vi "Historial de coordenadas.vi"(10 "Array":string[](array[string])) -> ()   [LabVIEW 2021]
panel:
  # "Lectura del arreglo de los cambios del setpoint"
  # "Elaborado por: Rodríguez Corona Ernesto \n04 de marzo del 2022"
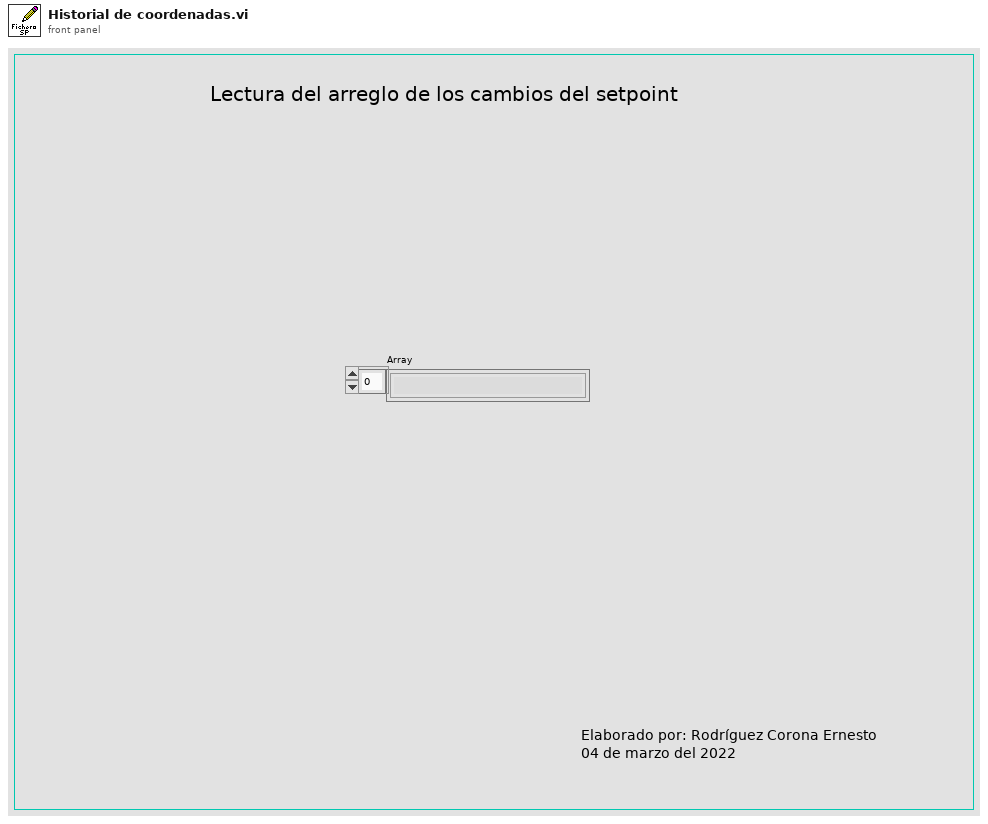
[diagram p1: front panel]
types:
  T1 = enum16{"open", "replace", "create", "open or create", "replace or create", "replace or create with confirmation"}
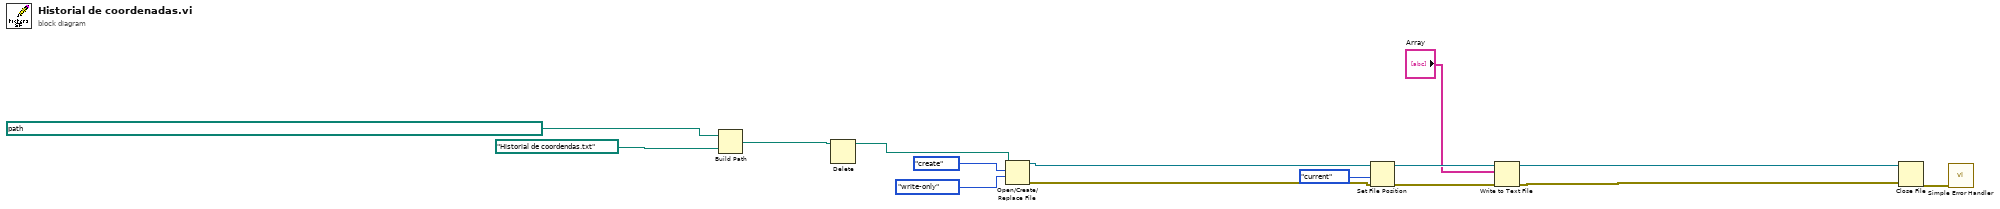
[diagram p0: block diagram]
diagram:
  n1 = Build Path(base path=path "C:/Users/netit/Desktop/Archivos Escolares/UTT/Séptimo Cuatrimestre/Baymax/Programación/Almacenamiento de historiales", name or relative path=path "Historial de coordendas.txt") -> (appended path=w7:path)
  n2 = Delete(path (use dialog)=w7) -> (deleted path=w6:path)  [unwired: 4 in, 2 out]
  n3 = Open/Create/Replace File(file path (use dialog)=w6, operation (0:open)=T1."create", access (0:read/write)=enum16{"read/write", "read-only", "write-only"}."write-only") -> (refnum out=w11:refnum<file>, error out=w10:errorcluster)  [unwired: 3 in, 1 out]
  n4 = Set File Position(refnum=w11, from (0:start)=enum16{"start", "end", "current"}."current", error in=w10) -> (refnum out=w4:refnum<file>, error out=w3:errorcluster)  [unwired: 1 in]
  n5 = Write to Text File(file (use dialog)=w4, text="Array", error in=w3) -> (refnum out=w14:refnum<file>, error out=w15:errorcluster)  [unwired: 1 in, 1 out]
  n6 = Close File(refnum=w14, error in=w15) -> (error out=w13:errorcluster)  [unwired: 1 out]
  n7 = call <vilib>:"Simple Error Handler.vi"("error in (no error)"=w13) -> ()  [unwired: 4 in, 5 out]
